vi "Compressor With Cylinder.vi"() -> ()   [LabVIEW 2023]
doc: "Compressor with Cylinder \n\nThis example shows how to control a compressor, extend and retract a cylinder, and optionally use a limit switch to retract automatically.\n\nThis example works with the PCM (Pneumatic Control Module) communicating with the roboRIO over CAN bus. The PCM must also be supplied with 12V DC from the PDP (Power Distribution Panel).\n\nThe Compressor, Pressure Switch, and Solenoids are all wired to the PCM \n\nThe Limit Switch is wired to DIO 9. It causes the cylinder to retract when the Auto Retract button is pressed.\n\nRefer to the Pneumatics Manual for air connections. Your pneumatics setup should include a compressor, pressure switch, tank, regulator, valve, flow controls, cylinder, plug valve, etc.\n\nTo run this example you should have a pneumatic system with air pressure connected to the P input on the SMC double solenoid valve. The A output of the valve should be connected via a flow control to the backend of a cylinder. The B output of the valve should be connected via a flow control to the frontend of a cylinder. When the cylinder is extended, it should physically depress the Limit Switch.\n\nWith the VI running, pressing the Extend button will push the cylinder shaft out, and pressing the Retract button will pull it back. Notice that the Extend and Retract buttons have their Mechanical Action set to Latch When Pressed. This means they stay pressed (ON) until they are read by the program, then they return to the OFF position. This works because once the SMC solenoid valve is pulled one direction, it stays in that position until it is pulled in the opposite direction - it only needs to be momentarily energized. The Auto Retract button can be used to make the cylinder return automatically. With the Auto Retract button ON, pressing the Extend button will push the cylinder out, and it will retract when it hits the limit switch.\n\nThis example expects a USB cable connected from your development PC to the Type B USB Jack (next to the power input) on the roboRIO.\n\nThis example expects the Driver Station to be running."
uses:
  <vilib>/Rock Robotics/WPI/Solenoid/WPI_SolenoidChannel.ctl
  <vilib>/Rock Robotics/WPI/Solenoid/WPI_SolenoidValue.ctl
  <vilib>/Rock Robotics/WPI/Solenoid/WPI_SolenoidOpenDouble.vi
  <vilib>/Rock Robotics/WPI/Solenoid/WPI_SolenoidSetEnum.vi
panel:
  in  "Compressor stop":bool
  in  "Lift Down":bool
  in  "Lift Up":bool
  in  "Lift  Down":T1=enum."Solenoid 3"
  in  "Lift Up":T1=enum."Solenoid 2"
  in  "Select a PD device by clicking on the image below":u16(ring) items=["CTRE Pneumatic Module", "REV Pneumatics Hub"]
  out "Compressor Running":bool
  in  "Lock In":bool
  in  "Loick In":T1
  in  "Lock Out":T1=enum."Solenoid 1"
  out "Compressor Monitoring":bool
  in  "stop":bool
  in  "Lock Out":bool
  # "Set these inputs before running."
  # "roboRIO Wiring Diagram"
  # "when extended, the cylinder should depress this"
  # "Limit\nSwitch"
  # "These can be set while running."
  # "Output information."
  # "COM"
  # "NC"
  # "NO"
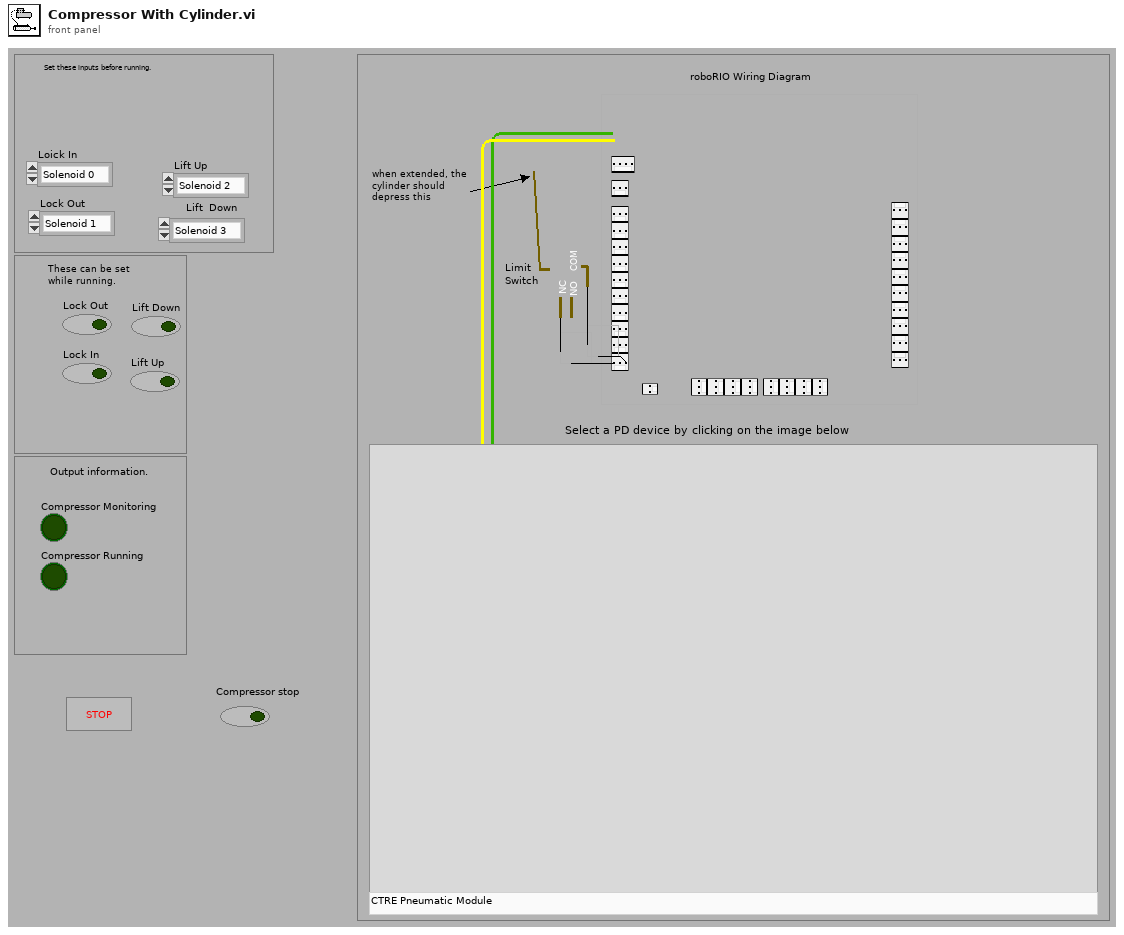
[diagram p1: front panel]
types:
  T1 = typedef "WPI_SolenoidChannel.ctl" = enum8{"Solenoid 0", "Solenoid 1", "Solenoid 2", "Solenoid 3", "Solenoid 4", "Solenoid 5", "Solenoid 6", "Solenoid 7", "Solenoid 8", "Solenoid 9", "Solenoid 10", "Solenoid 11", "Solenoid 12", "Solenoid 13", "Solenoid 14", "Solenoid 15", "Invalid"}
  T2 = typedef "WPI_CompressorDevRef.ctl" = cluster{"DevStatus":errorcluster, "Pneumatics Control Module":u8}
  T3 = typedef "WPI_SolenoidDevRef.ctl" = cluster{"DevStatus":errorcluster, "Pneumatics Control Module":u8, "Forward Solenoid Channel":T1, "Reverse Solenoid Channel":T1}
  T4 = typedef "WPI_SolenoidValue.ctl" = enum16{"Off", "On", "Forward", "Reverse"}
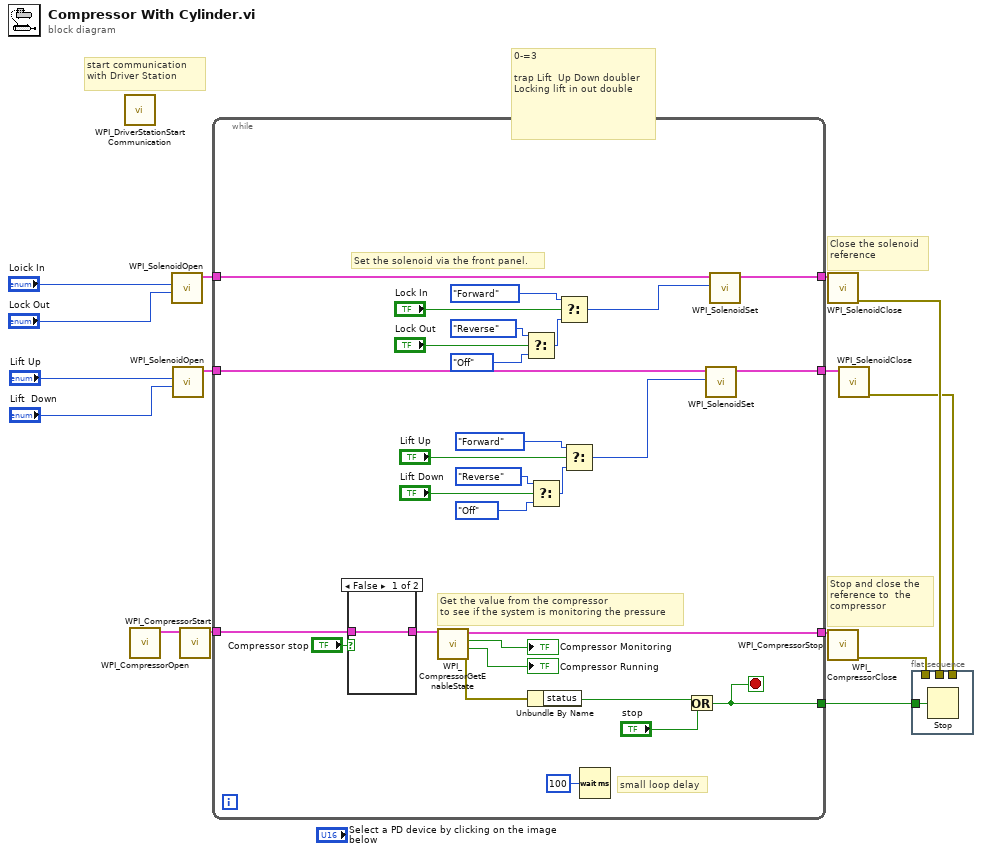
[diagram p0: block diagram]
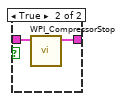
[diagram p2: hidden frame]
diagram:
  # "0-=3\n\ntrap Lift  Up Down doubler\nLocking lift in out double"
  # "Close the solenoid\nreference"
  # "start communication with Driver Station"
  # "Stop and close the reference to  the compressor"
  n1 = call <vilib>:"WPI_DriverStationStart Communication.vi"() -> ()  [unwired: 3 in, 9 out]
  n2 = call <vilib>:"WPI_CompressorOpen.vi"() -> ("CompressorDevRef"=w9:T2)  [unwired: 14 in, 1 out]
  n3 = call-poly <vilib>:"WPI_SolenoidOpen.vi"("Reverse Solenoid Channel"="Lock Out", "Forward Solenoid Channel"="Loick In") -> ("SolenoidDevRef"=w12:T3)  [unwired: 2 in, 7 out]
  n4 = call-poly <vilib>:"WPI_SolenoidOpen.vi"("Reverse Solenoid Channel"="Lift  Down", "Forward Solenoid Channel"="Lift Up") -> ("SolenoidDevRef"=w3:T3)  [unwired: 2 in, 7 out]
  n5 = call <vilib>:"WPI_CompressorStart.vi"("CompressorDevRef"=w9) -> ("CompressorDevRef"=w15:T2)  [unwired: 2 in, 8 out]
  n6 = while {
    tunnel: w15 -> [w18]
    tunnel: [w45] -> w14
    tunnel: [w43] -> w8
    tunnel: w12 -> [w38]
    tunnel: [w30] -> w13
    tunnel: w3 -> [w22]
    tunnel: [w20] -> w2
    stop <- w43 stop-if-true
    # "small loop delay"
    # "Get the value from the compressor \nto see if the system is monitoring the pressure"
    # "Set the solenoid via the front panel."
    n7 = case shown="False" "Compressor stop" {
      tunnel: [w46 w48] -> w19
      tunnel: w18 -> [w46 w47]
      frame False {
      }
      frame True {
        n8 = call <vilib>:"WPI_CompressorStop.vi"("CompressorDevRef"=w47) -> ("CompressorDevRef"=w48:T2)  [unwired: 9 in, 1 out]
      }
    }
    n9 = call <vilib>:"WPI_CompressorGetEnableState.vi"("CompressorDevRef"=w19) -> ("error out"=w41:errorcluster, "Compressor Running"=→"Compressor Running":bool, "Enabled"=→"Compressor Monitoring":bool, "CompressorDevRef"=w45:T2)  [unwired: 1 in, 6 out]
    n10 = Select(t=WPI_SolenoidValue."Reverse" ("Value"), s="Lock Out", f=WPI_SolenoidValue."Off" ("Value")) -> (s? t:f=w32:T4)
    n11 = Unbundle By Name(w41) -> ("status"=w40:bool)
    n12 = Select(t=WPI_SolenoidValue."Reverse" ("Value"), s="Lift Down", f=WPI_SolenoidValue."Off" ("Value")) -> (s? t:f=w27:T4)
    n13 = Select(t=WPI_SolenoidValue."Forward" ("Value"), s="Lock In", f=w32) -> (s? t:f=w29:T4)
    n14 = Select(t=WPI_SolenoidValue."Forward" ("Value"), s="Lift Up", f=w27) -> (s? t:f=w21:T4)
    n15 = Wait (ms)(milliseconds to wait=u32 100) -> ()  [unwired: 1 out]
    n16 = Or(x=w40, y="stop") -> (x .or. y?=w43:bool)
    n17 = call-poly <vilib>:"WPI_SolenoidSet.vi"("Value"=w21, "SolenoidDevRef"=w22) -> ("SolenoidDevRef"=w20:T3)  [unwired: 1 in, 8 out]
    n18 = call-poly <vilib>:"WPI_SolenoidSet.vi"("Value"=w29, "SolenoidDevRef"=w38) -> ("SolenoidDevRef"=w30:T3)  [unwired: 1 in, 8 out]
  }
  n19 = call <vilib>:"WPI_SolenoidClose.vi"("SolenoidDevRef"=w13) -> ("error out"=w6:errorcluster)  [unwired: 1 in, 9 out]
  n20 = call <vilib>:"WPI_CompressorStop.vi"("CompressorDevRef"=w14) -> ("CompressorDevRef"=w16:T2)  [unwired: 1 in, 9 out]
  n21 = call <vilib>:"WPI_CompressorClose.vi"("CompressorDevRef"=w16) -> ("error out"=w7:errorcluster)  [unwired: 1 in, 9 out]
  n22 = call <vilib>:"WPI_SolenoidClose.vi"("SolenoidDevRef"=w2) -> ("error out"=w1:errorcluster)  [unwired: 1 in, 9 out]
  n23 = flat-sequence {
    tunnel: w8 -> [w49]
    tunnel: w7 -> [_]
    tunnel: w6 -> [_]
    tunnel: w1 -> [_]
    frame #0 {
      n24 = Stop(stop? (T)=w49) -> ()
    }
  }
